vi "PS90_GetAxisState.vi"(8 "error in (no error)":errorcluster, 9 "Axis number":i32=1 min=0 max=9, 10 "Control unit ID":i32=1 min=1 max=10, 11 "DLOwis.lvclass":refnum<class "DLOwis.lvclass">) -> (0 "error out":errorcluster, 1 "Axis state":i32, 3 "DLOwis.lvclass":refnum<class "DLOwis.lvclass">)   [LabVIEW 2019, in "DLOwis.lvclass"]
doc: "PS90_GetAxisState.vi, created: 18.10.2006 alex; last change: 19.07.2016 alex;\n\n<B>FUNCTION:</B> \n\nRead axis state.\n----------------------------------------------------------------------------------------\n<B>INPUT:</B>\n[I32] <B>Control unit ID:</B> control unit index. (Default=1, Range=1...10) \n[I32] <B>Axis number:</B> axis number. (Default=1, Range=0...9)\n0 - read state of all axes,\n1...9 - read state of an axis. \n[CLU] <B>error in</B>\n----------------------------------------------------------------------------------------\n<B>OUTPUT:</B>\n[I32] <B>Axis state:</B> state of an axis or all axes.\nAxis number = 0 (all axes)\n0 - any axis is not active,\n1 - any axis is not initialized,\n2 - any axis is switch off,\n3 - all axes are active and initialized and switched on.\nAxis number = 1...9 (an axis)\n0 - axis is not active,\n1 - axis is not initialized,\n2 - axis is switched off,\n3 - axis is active and initialized and switched on.\n[CLU] <B>error out</B>\n----------------------------------------------------------------------------------------\n<B>SUB-VIs:</B>\nPS90_GetReadError.vi\n----------------------------------------------------------------------------------------\n<B>EXT-Calls:</B>\nps90.dll (V2.00)\n----------------------------------------------------------------------------------------"
uses:
  DLOwis.lvclass
  C:/Dev/TRANCON/Classes/Delay Line/DelayLine.lvclass
  DelayLine.lvclass/DelayLine.ctl
  DelayLine.lvclass
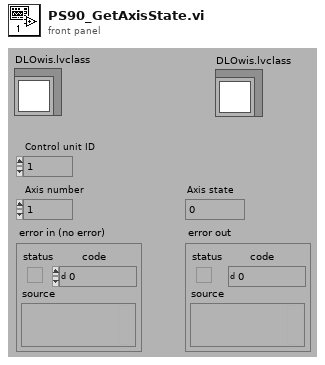
[diagram p1: front panel]
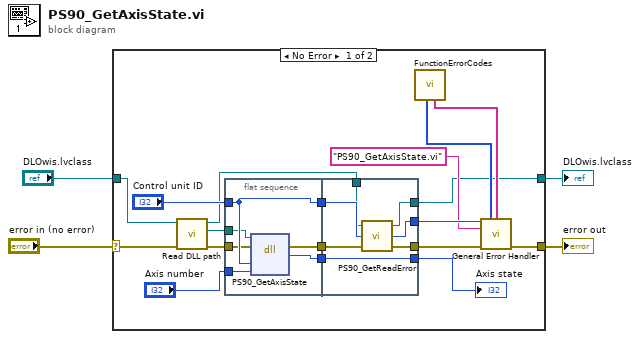
[diagram p0: block diagram]
diagram:
  n1 = case shown="No Error" "error in (no error)" {
    selector: "error in (no error)" -> [w14 w37]
    tunnel: [w21 w37] -> w4
    tunnel: [w7 w36] -> w2
    tunnel: "DLOwis.lvclass" -> [w13 w36]
    frame No Error {
      n2 = call "Read DLL path.vi"("error in (no error)"=w14, "DelayLine in"=w13) -> ("error out"=w12:errorcluster, "DLL path"=w5:path, "DelayLine out"=w8:refnum<class "DLOwis.lvclass">)  [unwired: 7 in]
      n3 = flat-sequence {
        tunnel: "Control unit ID" -> [w28]
        tunnel: [w28] -> w11
        tunnel: [w27] -> w10
        tunnel: "Axis number" -> [w26]
        tunnel: w12 -> [w25]
        tunnel: [w24] -> w9
        tunnel: w5 -> [w23]
        tunnel: w11 -> [w35]
        tunnel: [w33] -> w20
        tunnel: w10 -> [w33]
        tunnel: [w34] -> w19
        tunnel: w9 -> [w32]
        tunnel: w8 -> [w31]
        tunnel: [w30] -> w7
        tunnel: [w29] -> w6
        frame #0 {
          n4 = dll-call lib="C:/Dev/TRANCON/DLL/ps90.dll" fn="PS90_GetAxisState" label="PS90_Get\nAxisState"(path in=w23, error in=w25, "Index"=w28, "AxisNr"=w26) -> (error out=w24:errorcluster, "Rückgabetyp"=w27:i32)  [unwired: 3 in, 1 out]
        }
        frame #1 {
          n5 = call "PS90_GetReadError.vi"("error in (no error)"=w32, "Control unit ID"=w35, "DLOwis.lvclass"=w31) -> ("error IO"=w29:errorcluster, "Read error"=w34:i32, "DLOwis.lvclass"=w30:refnum<class "DLOwis.lvclass">)
        }
      }
      n6 = call "FunctionErrorCodes.vi"() -> ("[user-defined codes]"=w16:i32[], "[user-defined descriptions]"=w15:string[])  [unwired: 8 in]
      n7 = call <vilib>:"General Error Handler.vi"("[error code] (0)"=w19, "[user-defined codes]"=w16, "[user-defined descriptions]"=w15, "[error source] (\" \")"="PS90_GetAxisState.vi" ("[error source] (\" \")"), "error in (no error)"=w6) -> ("error out"=w21:errorcluster)  [unwired: 6 in, 4 out]
      "Axis state" <- w20
    }
    frame Error {
    }
  }
  "error out" <- w4
  "DLOwis.lvclass" <- w2
